vi "Start Acquiring.vi"(6 "wait for reply (T)":bool=TRUE, 8 "error in (no error)":errorcluster) -> (0 "error out":errorcluster, 1 "timed out?":bool, 2 "Reply Payload":T1)   [LabVIEW 2020, in "Acquisition.lvlib"]
doc: "<b>Note</b>: This VI was renamed by the DQMH Rename Event utility. Make sure the VI Description is updated to reflect the new event name, then delete this comment.\n\nRequests Acquisition Module to start acquiring.\n_____\nCreated using Delacor QMH Event Scripter 4.1.0.78.\n_____\nBased on DQMH Project Template 6.0.0.91."
uses:
  Acquisition.lvlib
  Start Acquiring (Reply Payload)--cluster.ctl
  Start Acquiring Argument--cluster.ctl
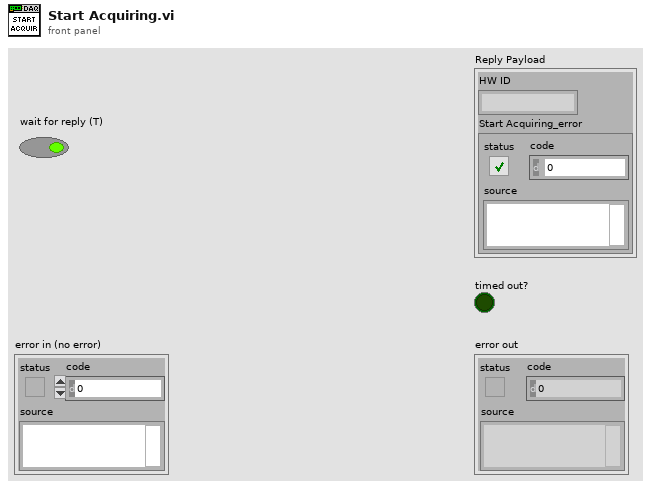
[diagram p1: front panel]
types:
  T1 = typedef "Acquisition.lvlib/Start Acquiring (Reply Payload)--cluster.ctl" = cluster{"HW ID":string, "Start Acquiring_error":errorcluster}
  T2 = typedef "Acquisition.lvlib/Request Events--cluster.ctl" = cluster{"Stop Module":refnum<user-event>, "Show Panel":refnum<user-event>, "Hide Panel":refnum<user-event>, "Get Module Execution Status":refnum<user-event>, "Show Diagram":refnum<user-event>, "Stop Acquiring":refnum<user-event>, "Wakeup Helper Loop":refnum<user-event>, "Change Settings":refnum<user-event>, "Calibrate DAQ":refnum<user-event>, "Start Acquiring":refnum<user-event>}
  T3 = typedef "Acquisition.lvlib/Start Acquiring Argument--cluster.ctl" = cluster{"Wait Notifier":refnum<notifier>, "wait for reply":bool}
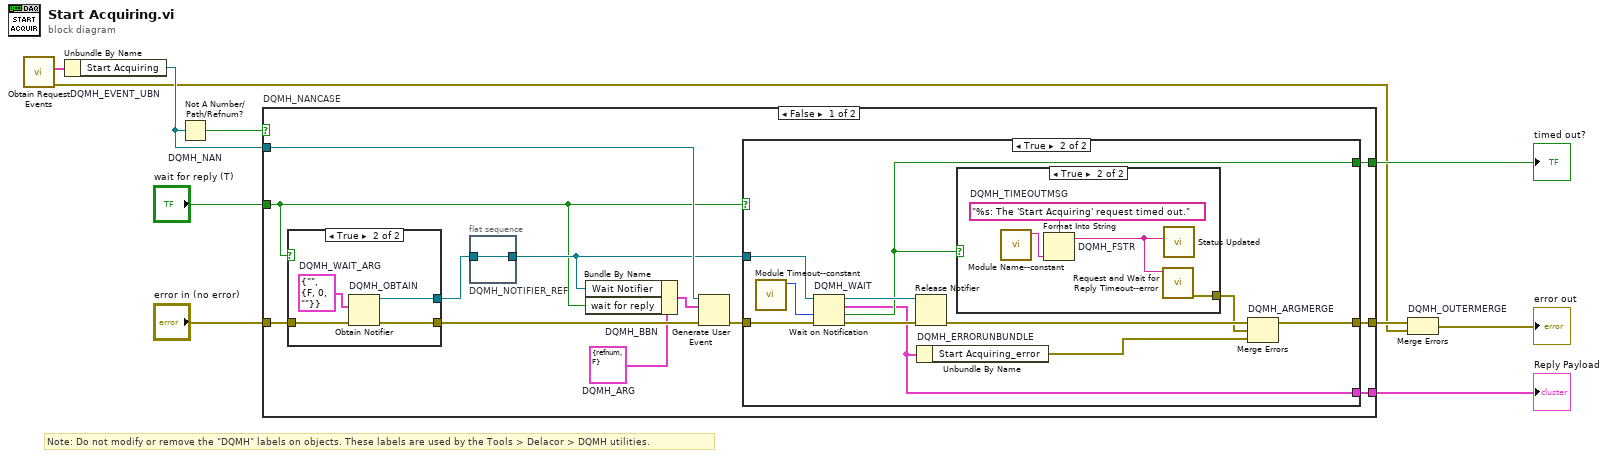
[diagram p0: block diagram]
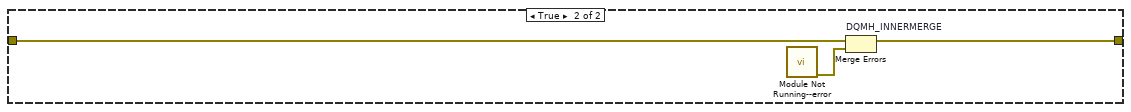
[diagram p5: hidden frame]
diagram:
  # "Note: Do not modify or remove the \"DQMH\" labels on objects. These labels are used by the Tools > Delacor > DQMH utilities."
  n1 = call "Obtain Request Events.vi"() -> ("error out"=w3:errorcluster, "Acquisition Request Events"=w2:T2)  [unwired: 10 in]
  n2 = Unbundle By Name "DQMH_EVENT_UBN"(w2) -> ("Start Acquiring"=w5:refnum<user-event>)
  n3 = Not A Number/Path/Refnum? "DQMH_NAN"(number/path/refnum=w5) -> (NaN/Path/Refnum?=w6:bool)
  n4 = case "DQMH_NANCASE" shown="False" w6 {
    tunnel: "error in (no error)" -> [w22 w47]
    tunnel: w5 -> [w20 _]
    tunnel: [w17 w46] -> w7
    tunnel: [w18 _] -> w9
    tunnel: "wait for reply (T)" -> [w12 _]
    tunnel: [w13 _] -> w1
    frame False {
      w11 = T3 {"Wait Notifier"=refnum, "wait for reply"=FALSE}  # DQMH_ARG
      n5 = case shown="True" w12 {
        tunnel: w22 -> [w40 w44]
        tunnel: [w40 w43] -> w19
        tunnel: [_ w42] -> w15
        frame False {
        }
        frame True {
          w41 = T1 {"HW ID"="", "Start Acquiring_error"={"status"=FALSE, "code"=0, "source"=""}}  # DQMH_WAIT_ARG
          n6 = Obtain Notifier "DQMH_OBTAIN"(notification data type=w41, error in (no error)=w44) -> (notifier out=w42:refnum<notifier>, error out=w43:errorcluster)  [unwired: 2 in, 1 out]
        }
      }
      n7 = flat-sequence "DQMH_NOTIFIER_REF" {
        tunnel: w15 -> [w23]
        tunnel: [w23] -> w14
        frame #0 {
        }
      }
      n8 = Bundle By Name "DQMH_BBN"(cluster=w11, "Wait Notifier"=w14, "wait for reply"=w12) -> (w16:T3)
      n9 = Generate User Event(user event=w20, event data cluster=w16, error in=w19) -> (error out=w21:errorcluster)  [unwired: 1 in, 1 out]
      n10 = case shown="True" w12 {
        tunnel: w21 -> [w24 w35]
        tunnel: w14 -> [_ w34]
        tunnel: [_ w32] -> w18
        tunnel: [w24 w31] -> w17
        tunnel: [_ w27] -> w13
        frame False {
        }
        frame True {
          n11 = call "Module Timeout--constant.vi"() -> ("Module Timeout"=w30:i32)  [unwired: 11 in]
          n12 = Wait on Notification "DQMH_WAIT"(notifier=w34, timeout in ms (-1)=w30, error in (no error)=w35) -> (notifier out=w33:refnum<notifier>, notification=w27:T1, timed out?=w32:bool, error out=w29:errorcluster)  [unwired: 1 in]
          n13 = Release Notifier(notifier=w33, error in (no error)=w29) -> (error out=w28:errorcluster)  [unwired: 1 in, 2 out]
          n14 = Unbundle By Name "DQMH_ERRORUNBUNDLE"(w27) -> ("Start Acquiring_error"=w26:errorcluster)
          n15 = case shown="True" w32 {
            tunnel: [_ w36] -> w25
            frame False {
            }
            frame True {
              w39 = "%s: The 'Start Acquiring' request timed out."  # DQMH_TIMEOUTMSG
              n16 = call "Module Name--constant.vi"() -> ("Module Name"=w38:string)  [unwired: 11 in]
              n17 = Format Into String "DQMH_FSTR"(format string=w39, w38) -> (resulting string=w37:string)  [unwired: 2 in, 1 out]
              n18 = call "Request and Wait for Reply Timeout--error.vi"("Error Message"=w37) -> ("error out"=w36:errorcluster)  [unwired: 10 in]
              n19 = call "Status Updated.vi"("Status"=w37) -> ()  [unwired: 10 in, 1 out]
            }
          }
          n20 = Merge Errors "DQMH_ARGMERGE"(w28, w25, w26) -> (w31:errorcluster)
        }
      }
    }
    frame True {
      n21 = call "Module Not Running--error.vi"() -> ("error out"=w45:errorcluster)  [unwired: 11 in]
      n22 = Merge Errors "DQMH_INNERMERGE"(w47, w45) -> (w46:errorcluster)
    }
  }
  "timed out?" <- w9
  "Reply Payload" <- w1
  n23 = Merge Errors "DQMH_OUTERMERGE"(w7, w3) -> (→"error out":errorcluster)
